vi "ICNC Update Speed.vi"(8 "error in (no error)":errorcluster caption="entrée d'erreur (pas d'erreur)", 10 "NewFrenquency":u32, 11 "Axe":u32) -> (0 "error out":errorcluster caption="sortie d'erreur", 3 "function return":u32)   [LabVIEW 2012, in "ICNC2.lvlib"]
doc: "DWORD ICNC_UpdateSpeed( DWORD Axe,\n DWORD NewFrenquency);"
uses:
  <userlib>/ICNC/ICNC2.lvlib
  <userlib>/ICNC/ICNC2.dll
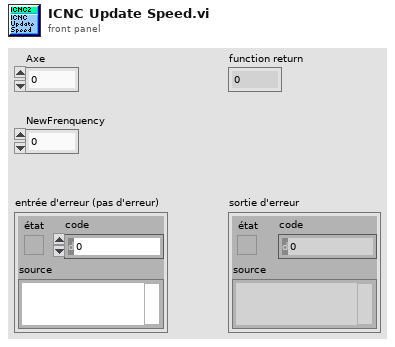
[diagram p1: front panel]
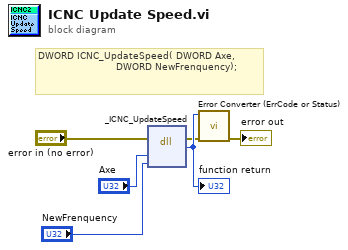
[diagram p0: block diagram]
diagram:
  # "DWORD ICNC_UpdateSpeed( DWORD Axe,\n                          DWORD NewFrenquency);"
  n1 = dll-call lib="C:/Program Files (x86)/National Instruments/LabVIEW 2012/user.lib/ICNC/ICNC2.*" fn="_ICNC_UpdateSpeed"(error in="error in (no error)", "Axe"="Axe", "NewFrenquency"="NewFrenquency") -> (error out=w2:errorcluster, w6:u32)  [unwired: 4 in, 1 out]
  "function return" <- w6
  n2 = call <userlib>:"Error Converter (ErrCode or Status).vi"("error in (no error)"=w2, "error code"=w6) -> ("error out"=→"error out":errorcluster)  [unwired: 9 in]
